vi "MathOptim-Fit Stats.vi"(0 "Y":dbl[](array[numeric]), 5 "Yfit":dbl[](array[numeric]), 7 "Num params":i32) -> (4 "SSE":dbl, 6 "R2":dbl, 8 "adjusted R2":dbl, 10 "summary":string)   [LabVIEW 2020]
uses:
  <vilib>/Analysis/baseanly.llb/Mean (DBL).vi
  <vilib>/Analysis/NI_AALBase.lvlib
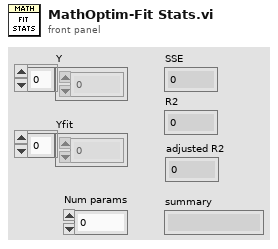
[diagram p1: front panel]
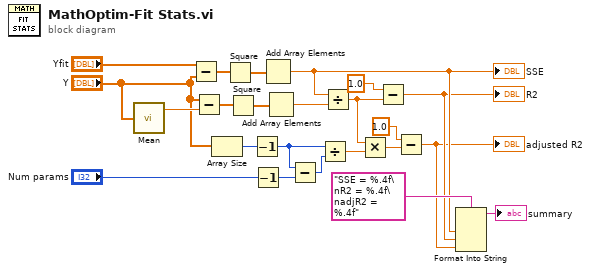
[diagram p0: block diagram]
diagram:
  n1 = call-poly <vilib>:"Mean.vi"("X"="Y") -> ("mean"=w18:dbl)  [unwired: 1 out]
  n2 = Subtract(x="Yfit", y="Y") -> (x-y=w22:dbl[])
  n3 = Subtract(x="Y", y=w18) -> (x-y=w20:dbl[])
  n4 = Array Size(array="Y") -> (size(s)=w14:i32)
  n5 = Square(x=w22) -> (x^2=w21:dbl[])
  n6 = Square(x=w20) -> (x^2=w19:dbl[])
  n7 = Decrement(x=w14) -> (x-1=w11:i32)
  n8 = Decrement(x="Num params") -> (x-1=w12:i32)
  n9 = Add Array Elements(numeric array=w21) -> (sum=w4:dbl)
  "SSE" <- w4
  n10 = Add Array Elements(numeric array=w19) -> (sum=w17:dbl)
  n11 = Subtract(x=w11, y=w12) -> (x-y=w10:i32)
  n12 = Divide(x=w11, y=w10) -> (x/y=w9:dbl)
  n13 = Divide(x=w4, y=w17) -> (x/y=w8:dbl)
  n14 = Multiply(x=w8, y=w9) -> (x*y=w7:dbl)
  n15 = Subtract(x=1.0, y=w8) -> (x-y=w3:dbl)
  "R2" <- w3
  n16 = Subtract(x=1.0, y=w7) -> (x-y=w2:dbl)
  "adjusted R2" <- w2
  n17 = Format Into String(format string="SSE = %.4f\nR2 = %.4f\nadjR2 = %.4f", w4, w3, w2) -> (resulting string=→"summary":string)  [unwired: 2 in, 1 out]
